vi "PDC_SetShutterSpeedFps.vi"(8 "error in (no error)":errorcluster, 9 "Fps":u32, 10 "ChildNo":u32, 11 "DeviceNo":u32) -> (0 "error out":errorcluster, 3 "ReturnValue":u32, 4 "ErrorCode":u32)   [LabVIEW 2015]
doc: "This VI sets the shutter speed of the specified child device."
uses:
  PDCLIB.dll
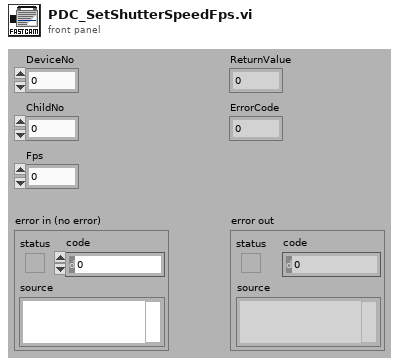
[diagram p1: front panel]
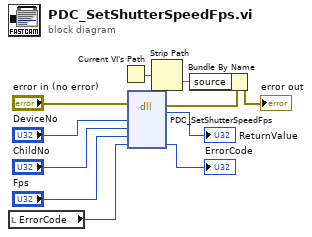
[diagram p0: block diagram]
diagram:
  n1 = local read "ErrorCode"() -> (w8:u32)
  n2 = Current VI's Path() -> (path=w3:path)
  n3 = dll-call lib="PDCLIB.dll" fn="PDC_SetShutterSpeedFps"(error in="error in (no error)", "nDeviceNo"="DeviceNo", "nChildNo"="ChildNo", "nFps"="Fps", "pErrorCode"=w8) -> (error out=w2:errorcluster, "return type"=→"ReturnValue":u32, "pErrorCode"=→"ErrorCode":u32)  [unwired: 5 in, 1 out]
  n4 = Strip Path(path=w3) -> (name=w4:string)  [unwired: 1 out]
  n5 = Bundle By Name(cluster=w2, "source"=w4) -> (→"error out":errorcluster)
